vi "Untitled 1.vi"() -> ()   [LabVIEW 2014]
uses:
  <vilib>/measure/NI_MABase.lvlib
panel:
  out "String":string
  in  "sampling info":cluster{"Fs":dbl, "#s":dbl}
  in  "duty cycle(%)":dbl format="%.2g"
  in  "offset":dbl format="%.2g"
  in  "Enum":T1(ring)
  in  "stop":bool
  in  "reset":bool
  in  "faza":dbl format="%.2g"
  in  "amplitudine":dbl format="%.2g"
  in  "frecventa":dbl format="%.2g"
  out "error out":errorcluster
  in  "error in (no error)":errorcluster
  out "Waveform Graph":waveform(dbl)(graph)
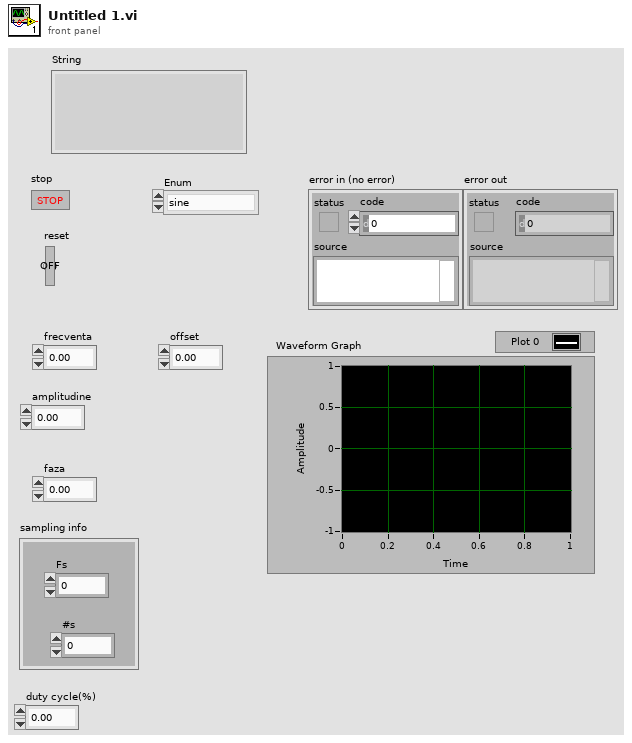
[diagram p1: front panel]
types:
  T1 = enum16{"sine", "triangle wave", "square wave", "sawtooth wave"}
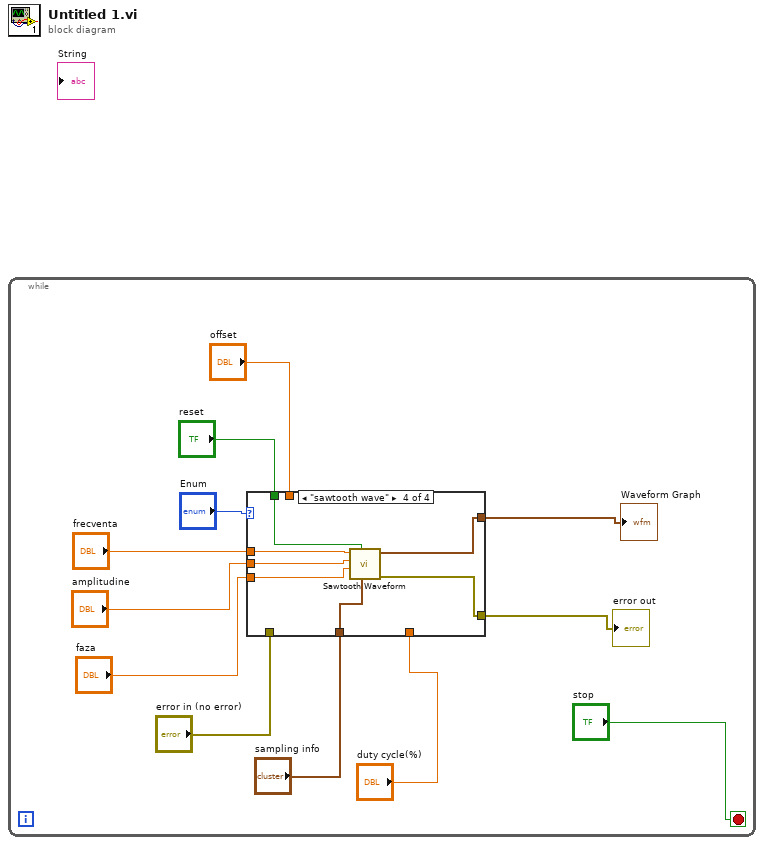
[diagram p0: block diagram]
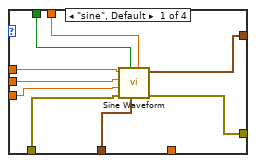
[diagram p2: hidden frame]
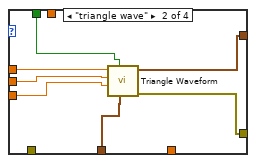
[diagram p3: hidden frame]
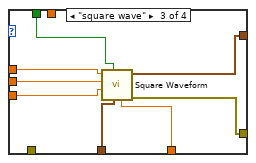
[diagram p4: hidden frame]
diagram:
  n1 = while {
    stop <- "stop" stop-if-true
    n2 = case shown="\"sawtooth wave\"" "Enum" {
      tunnel: "reset" -> [w21 w28 w36 w43]
      tunnel: "offset" -> [w20 _ _ _]
      tunnel: "frecventa" -> [w19 w24 w31 w39]
      tunnel: "amplitudine" -> [w18 w23 w30 w38]
      tunnel: "faza" -> [w17 w22 w29 w37]
      tunnel: "error in (no error)" -> [w16 _ _ _]
      tunnel: [w15 w27 w33 w40] -> w5
      tunnel: [w14 w26 w34 w41] -> w4
      tunnel: "sampling info" -> [w13 w25 w32 w42]
      tunnel: "duty cycle(%)" -> [_ _ w35 _]
      frame "sine", Default {
        n3 = call <vilib>:"Sine Waveform.vi"("offset"=w20, "sampling info"=w13, "reset signal"=w21, "error in (no error)"=w16, "phase"=w17, "amplitude"=w18, "frequency"=w19) -> ("error out"=w14:errorcluster, "signal out"=w15:waveform(dbl))  [unwired: 3 in]
      }
      frame "triangle wave" {
        n4 = call <vilib>:"Triangle Waveform.vi"("sampling info"=w25, "reset signal"=w28, "phase"=w22, "amplitude"=w23, "frequency"=w24) -> ("error out"=w26:errorcluster, "signal out"=w27:waveform(dbl))  [unwired: 5 in]
      }
      frame "square wave" {
        n5 = call <vilib>:"Square Waveform.vi"("duty cycle (%)"=w35, "sampling info"=w32, "reset signal"=w36, "phase"=w29, "amplitude"=w30, "frequency"=w31) -> ("error out"=w34:errorcluster, "signal out"=w33:waveform(dbl))  [unwired: 4 in]
      }
      frame "sawtooth wave" {
        n6 = call <vilib>:"Sawtooth Waveform.vi"("sampling info"=w42, "reset signal"=w43, "phase"=w37, "amplitude"=w38, "frequency"=w39) -> ("error out"=w41:errorcluster, "signal out"=w40:waveform(dbl))  [unwired: 5 in]
      }
    }
    "Waveform Graph" <- w5
    "error out" <- w4
  }
